vi "weekly graph.vi"(6 "country index":u16, 7 "SA data":T1, 8 "Countries (in)":string[](array[string]), 9 "US data":T1, 10 "deaths CSV":string[][](array[string]), 11 "cases CSV":string[][](array[string])) -> ()   [LabVIEW 2019]
panel:
  out "XY Graph":cluster{"array index":i32[], "weekly":u32[]}(graph)
  in  "Data":u16(ring) items=["new cases per day", "new deaths per day"]
  in  "Country 1":u16(ring) items=["Afghanistan", "Albania", "Algeria", "Andorra", "Angola", "Antigua and Barbuda", "Argentina", "Armenia", "Australia, Australian Capital Territory", "Australia, New South Wales", "Australia, Northern Territory", "Australia, Queensland", "Australia, South Australia", "Australia, Tasmania", "Australia, Victoria", "Australia, Western Australia", "Austria", "Azerbaijan", "Bahamas", "Bahrain", "Bangladesh", "Barbados", "Belarus", "Belgium", "Benin", "Bhutan", "Bolivia", "Bosnia and Herzegovina", "Brazil", "Brunei", "Bulgaria", "Burkina Faso", "Cabo Verde", "Cambodia", "Cameroon", "Canada, Alberta", "Canada, British Columbia", "Canada, Grand Princess", "Canada, Manitoba", "Canada, New Brunswick", "Canada, Newfoundland and Labrador", "Canada, Nova Scotia", "Canada, Ontario", "Canada, Prince Edward Island", "Canada, Quebec", "Canada, Saskatchewan", "Central African Republic", "Chad", "Chile", "China, Anhui", "China, Beijing", "China, Chongqing", "China, Fujian", "China, Gansu", "China, Guangdong", "China, Guangxi", "China, Guizhou", "China, Hainan", "China, Hebei", "China, Heilongjiang", "China, Henan", "China, Hong Kong", "China, Hubei", "China, Hunan", "China, Inner Mongolia", "China, Jiangsu", "China, Jiangxi", "China, Jilin", "China, Liaoning", "China, Macau", "China, Ningxia", "China, Qinghai", "China, Shaanxi", "China, Shandong", "China, Shanghai", "China, Shanxi", "China, Sichuan", "China, Tianjin", "China, Tibet", "China, Xinjiang", "China, Yunnan", "China, Zhejiang", "Colombia", "Congo (Brazzaville)", "Congo (Kinshasa)", "Costa Rica", "Cote d'Ivoire", "Croatia", "Diamond Princess", "Cuba", "Cyprus", "Czechia", "Denmark, Faroe Islands", "Denmark, Greenland", "Denmark", "Djibouti", "Dominican Republic", "Ecuador", "Egypt", "El Salvador", "Equatorial Guinea", "Eritrea", "Estonia", "Eswatini", "Ethiopia", "Fiji", "Finland", "France, French Guiana", "France, French Polynesia", "France, Guadeloupe", "France, Mayotte", "France, New Caledonia", "France, Reunion", "France, Saint Barthelemy", "France, St Martin", "France, Martinique", "France", "Gabon", "Gambia", "Georgia", "Germany", "Ghana", "Greece", "Guatemala", "Guinea", "Guyana", "Haiti", "Holy See", "Honduras", "Hungary", "Iceland", "India", "Indonesia", "Iran", "Iraq", "Ireland", "Israel", "Italy", "Jamaica", "Japan", "Jordan", "Kazakhstan", "Kenya", "Korea South", "Kuwait", "Kyrgyzstan", "Latvia", "Lebanon", "Liberia", "Liechtenstein", "Lithuania", "Luxembourg", "Madagascar", "Malaysia", "Maldives", "Malta", "Mauritania", "Mauritius", "Mexico", "Moldova", "Monaco", "Mongolia", "Montenegro", "Morocco", "Namibia", "Nepal", "Netherlands, Aruba", "Netherlands, Curacao", "Netherlands, Sint Maarten", "Netherlands", "New Zealand", "Nicaragua", "Niger", "Nigeria", "North Macedonia", "Norway", "Oman", "Pakistan", "Panama", "Papua New Guinea", "Paraguay", "Peru", "Philippines", "Poland", "Portugal", "Qatar", "Romania", "Russia", "Rwanda", "Saint Lucia", "Saint Vincent and the Grenadines", "San Marino", "Saudi Arabia", "Senegal", "Serbia", "Seychelles", "Singapore", "Slovakia", "Slovenia", "Somalia", "South Africa", "Spain", "Sri Lanka", "Sudan", "Suriname", "Sweden", "Switzerland", "Taiwan*", "Tanzania", "Thailand", "Togo", "Trinidad and Tobago", "Tunisia", "Turkey", "Uganda", "Ukraine", "United Arab Emirates", "United Kingdom, Bermuda", "United Kingdom, Cayman Islands", "United Kingdom, Channel Islands", "United Kingdom, Gibraltar", "United Kingdom, Isle of Man", "United Kingdom, Montserrat", "United Kingdom", "Uruguay", "US", "Uzbekistan", "Venezuela", "Vietnam", "Zambia", "Zimbabwe", "Canada, Diamond Princess", "Dominica", "Grenada", "Mozambique", "Syria", "Timor-Leste", "Belize", "Laos", "Libya", "West Bank and Gaza", "Guinea-Bissau", "Mali", "Saint Kitts and Nevis", "Canada, Northwest Territories", "Canada, Yukon", "Kosovo", "Burma", "United Kingdom, Anguilla", "United Kingdom, British Virgin Islands", "United Kingdom, Turks and Caicos Islands", "MS Zaandam", "Botswana", "Burundi", "Sierra Leone", "Netherlands, \"Bonaire Sint Eustatius and Saba\"", "Malawi", "United Kingdom, Falkland Islands (Malvinas)", "France, Saint Pierre and Miquelon", "South Sudan", "Western Sahara", "Sao Tome and Principe", "Yemen", "Comoros", "Tajikistan", "Lesotho", "Australia", "Western Europe", "Latin America", "Africa", "China", "US and Canada", "US - Northeast", "US - Midwest", "US - South", "US - West", "Scandinavia (excl Sweden)", "Global", "South Asia", "South East Asia", "East Asia", "Eastern Europe and Russia", "Middle East", "Central Asia", "Canada", "US excluding Northeast", "American Samoa", "Guam", "Northern Mariana Islands", "Puerto Rico", "Virgin Islands", "Alabama", "Alaska", "Arizona", "Arkansas", "California", "Colorado", "Connecticut", "Delaware", "Florida", "Georgia", "Hawaii", "Idaho", "Illinois", "Indiana", "Iowa", "Kansas", "Kentucky", "Louisiana", "Maine", "Maryland", "Massachusetts", "Michigan", "Minnesota", "Mississippi", "Missouri", "Montana", "Nebraska", "Nevada", "New Hampshire", "New Jersey", "New Mexico", "New York", "North Carolina", "North Dakota", "Ohio", "Oklahoma", "Oregon", "Pennsylvania", "Rhode Island", "South Carolina", "South Dakota", "Tennessee", "Texas", "Utah", "Vermont", "Virginia", "Washington", "West Virginia", "Wisconsin", "Wyoming", "SA, EC", "SA, FS", "SA, GP", "SA, KZN", "SA, LP", "SA, MP", "SA, NC", "SA, NW", "SA, WC"]
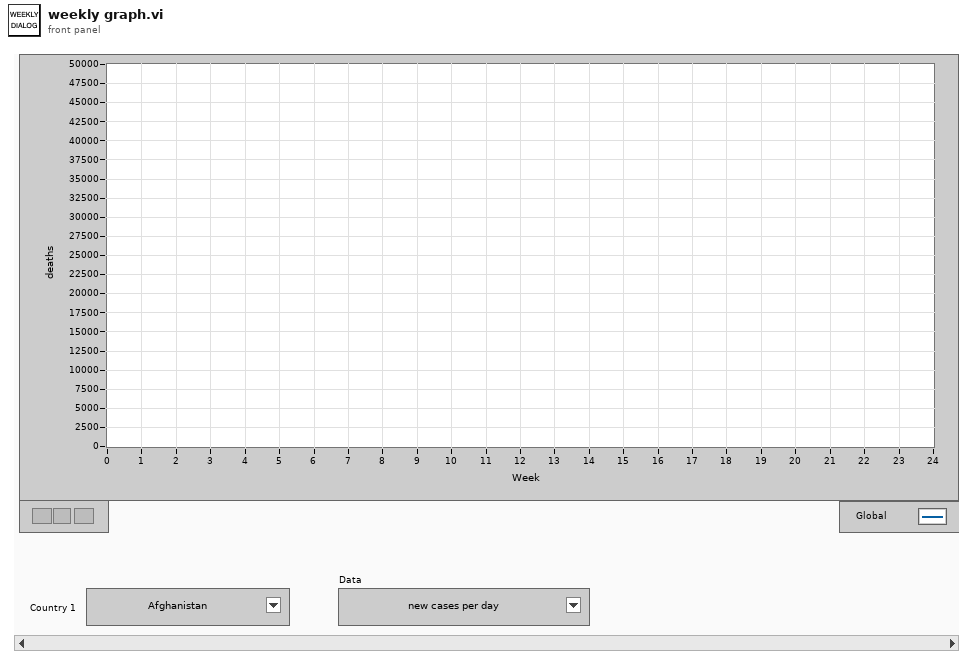
[diagram p1: front panel]
types:
  T1 = cluster{"cumulative deaths":i32[][], "deaths per day":i32[][], "case per day":i32[][], "cumulative cases":i32[][]}
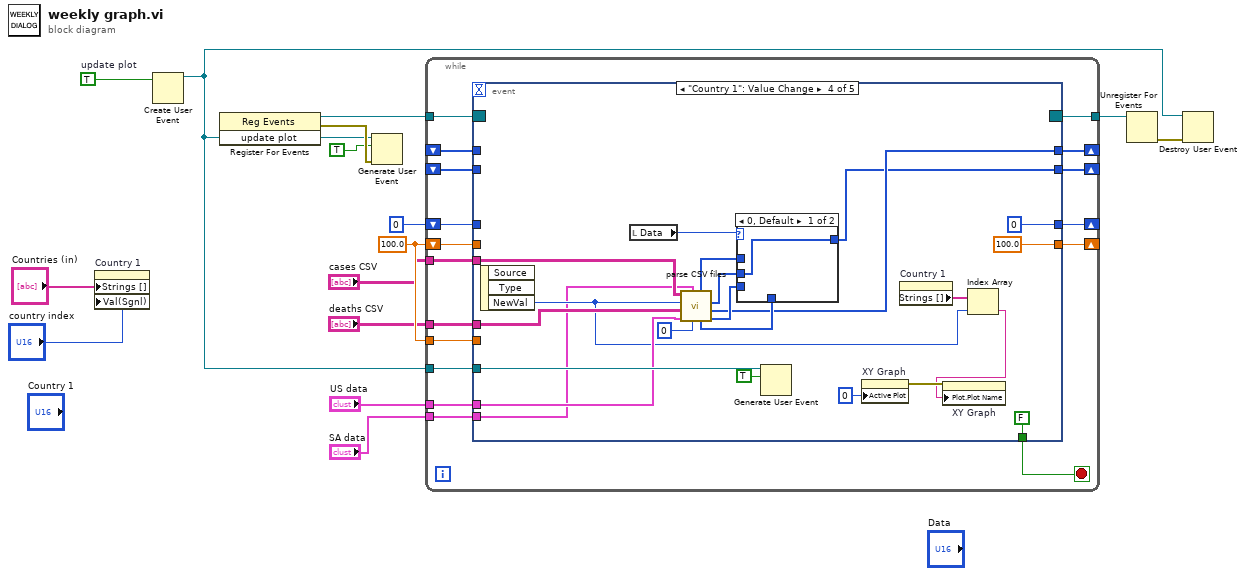
[diagram p0: block diagram]
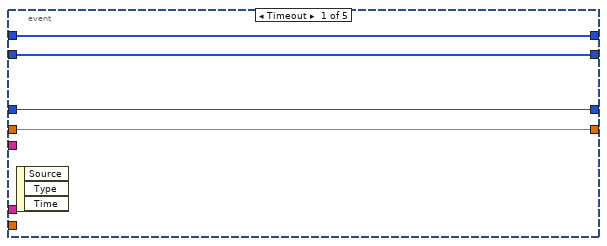
[diagram p2: hidden frame]
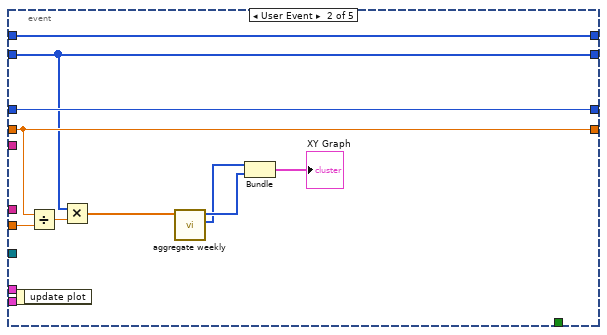
[diagram p3: hidden frame]
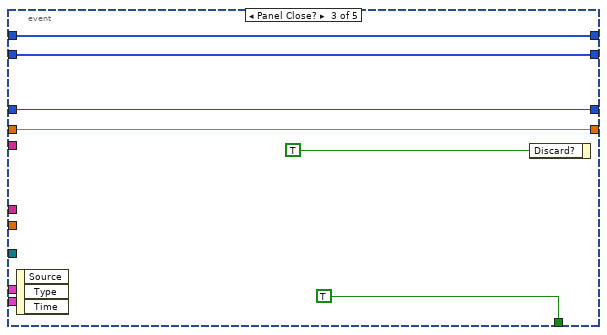
[diagram p4: hidden frame]
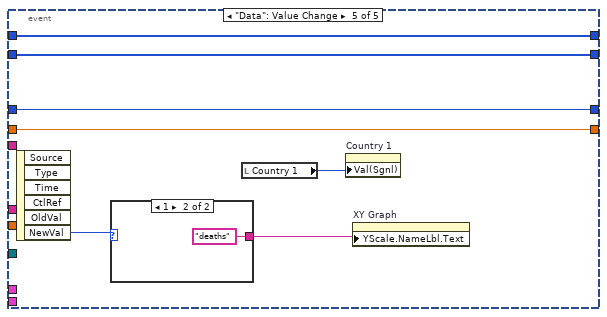
[diagram p6: hidden frame]
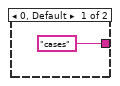
[diagram p7: hidden frame]
diagram:
  w11 = 100.0
  w13 = TRUE  # update plot
  n1 = property on="Country 1" class="Ring (strict)"("Strings []"="Countries (in)", "Val(Sgnl)"="country index") -> ()  [unwired: 2 in, 2 out]
  n2 = Create User Event(user event datatype=w13) -> (user event=w7:refnum<user-event>)  [unwired: 1 in, 1 out]
  n3 = register-events(w7) -> (reference out=w14:refnum<event-registration>, error out=w12:errorcluster)  [unwired: 2 in]
  n4 = Generate User Event(user event=w7, event data cluster=TRUE ("event data"), error in=w12) -> ()  [unwired: 1 in, 2 out]
  n5 = while {
    shift-right: [w30] -> _
    shift-left: _ -> [w32]
    shift-right: [w29] -> _
    shift-left: _ -> [w31]
    shift-right: [w27] -> _
    shift-left: 0 -> [w28]
    tunnel: w14 -> [w26]
    tunnel: w7 -> [w25]
    shift-right: [w23] -> _
    shift-left: w11 -> [w24]
    tunnel: w11 -> [w22]
    tunnel: [w20] -> w9
    tunnel: "cases CSV" -> [w19]
    tunnel: "deaths CSV" -> [w18]
    tunnel: "US data" -> [w17]
    tunnel: "SA data" -> [w16]
    stop <- w21 stop-if-true
    n6 = event shown="[3] \"Country 1\": Value Change" {
      selector: w26 -> [_ _ _ _ _]
      dyn-events: [_ _ _ _ _] -> w20
      timeout: _ -> [_ _ _ _ _]
      tunnel: w32 -> [w36 w39 w47 _ w79]
      tunnel: w31 -> [w35 w42 w52 _ w83]
      tunnel: [w36 w39 w47 w62 w79] -> w30
      tunnel: [w35 w42 w52 w61 w83] -> w29
      tunnel: w28 -> [w34 w44 w51 _ w82]
      tunnel: [w34 w44 w51 0 w82] -> w27
      tunnel: w25 -> [_ _ _ w71 _]
      tunnel: w24 -> [w33 w43 w50 _ w81]
      tunnel: [w33 w43 w50 100.0 w81] -> w23
      tunnel: w22 -> [_ w46 _ _ _]
      tunnel: [_ _ TRUE FALSE _] -> w21
      tunnel: w19 -> [_ _ _ w69 _]
      tunnel: w18 -> [_ _ _ w68 _]
      tunnel: w17 -> [_ _ _ w67 _]
      tunnel: w16 -> [_ _ _ w54 _]
      event Timeout {
        n7 = event-data() -> ()  [unwired: 1 in, 3 out]
      }
      event User Event {
        n8 = event-data() -> ()  [unwired: 1 in, 1 out]
        n9 = Divide(x=w43, y=w46) -> (x/y=w45:dbl)
        n10 = Multiply(x=w42, y=w45) -> (x*y=w41:dbl[])
        n11 = call "aggregate weekly.vi"("Array"=w41) -> ("array index"=w38:i32[], "weekly"=w40:u32[])  [unwired: 9 in]
        n12 = Bundle("array index"=w38, "weekly"=w40) -> (→"XY Graph":cluster{"array index":i32[], "weekly":u32[]})  [unwired: 1 in]
      }
      event Panel Close? {
        n13 = event-data() -> ()  [unwired: 1 in, 3 out]
        n14 = event-data("Discard?"=TRUE) -> ()  [unwired: 1 in, 1 out]
      }
      event "Country 1": Value Change {
        n15 = event-data() -> ("NewVal"=w56:u16)  [unwired: 1 in, 2 out]
        n16 = local read "Data"() -> (w53:u16)
        n17 = call "parse CSV files.vi"("threshold cases"=u32 0, "SA data"=w54, "US data"=w67, "deaths CSV"=w68, "country index"=w56, "cases CSV"=w69) -> ("new deaths per day"=w65:i32[], "days"=w62:i32[], "new cases per day"=w66:i32[], "cumulative cases"=w64:i32[], "cumulative deaths"=w63:i32[])  [unwired: 1 out]
        n18 = case shown="0, Default" w53 {
          tunnel: w66 -> [w75 _]
          tunnel: w65 -> [_ w76]
          tunnel: w64 -> [_ _]
          tunnel: w63 -> [_ _]
          tunnel: [w75 w76] -> w61
          frame 0, Default {
          }
          frame 1 {
          }
        }
        n19 = Generate User Event(user event=w71, event data cluster=TRUE ("event data")) -> ()  [unwired: 2 in, 2 out]
        n20 = property on="XY Graph" class="XYGraph (strict)"("Active Plot"=u32 0) -> (error out=w59:errorcluster)  [unwired: 2 in, 1 out]
        n21 = property on="Country 1" class="Ring (strict)"() -> ("Strings []"=w57:string[])  [unwired: 2 in, 2 out]
        n22 = Index Array(array=w57, index=w56) -> (element=w55:string)
        n23 = property on="XY Graph" class="XYGraph (strict)"(error in=w59, "Plot.Plot Name"=w55) -> ()  [unwired: 1 in, 2 out]
      }
      event "Data": Value Change {
        n24 = event-data() -> ("NewVal"=w78:u16)  [unwired: 1 in, 5 out]
        n25 = case shown="1" w78 {
          tunnel: ["cases" "deaths"] -> w77
          frame 0, Default {
          }
          frame 1 {
          }
        }
        n26 = local read "Country 1"() -> (w80:u16)
        n27 = property on="Country 1" class="Ring (strict)"("Val(Sgnl)"=w80) -> ()  [unwired: 2 in, 2 out]
        n28 = property on="XY Graph" class="XYGraph (strict)"("YScale.NameLbl.Text"=w77) -> ()  [unwired: 2 in, 2 out]
      }
    }
  }
  n29 = Unregister For Events(event registration refnum=w9) -> (error out=w8:errorcluster)  [unwired: 1 in]
  n30 = Destroy User Event(user event=w7, error in=w8) -> ()  [unwired: 1 out]
